vi "Open System Definition.vi"(8 "error in (no error)":errorcluster, 11 "System Definition File":path) -> (0 "error out":errorcluster, 2 "Embedded Data Logger":refnum<k39>, 3 "System Definiton":refnum<k39>)   [LabVIEW 2027, in "Embedded Data Logger Unit Tests.lvclass"]
uses:
  Embedded Data Logger Unit Tests.lvclass
  Embedded Data Logger Unit Tests.lvclass/Embedded Data Logger Unit Tests.ctl
  C:/NetCore/niveristand-embedded-data-logger-custom-device/Source/Tests/Unit/Open System Definition.vi/NationalInstruments.VeriStand.SystemDefinitionAPI
  NationalInstruments.VeriStand.SystemDefinitionAPI
  C:/NetCoreDLL/NationalInstruments.VeriStand.SystemDefinitionAPI.dll
  NetCoreDLL/NationalInstruments.VeriStand.SystemDefinitionAPI.dll
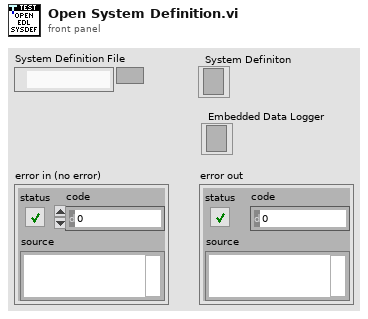
[diagram p1: front panel]
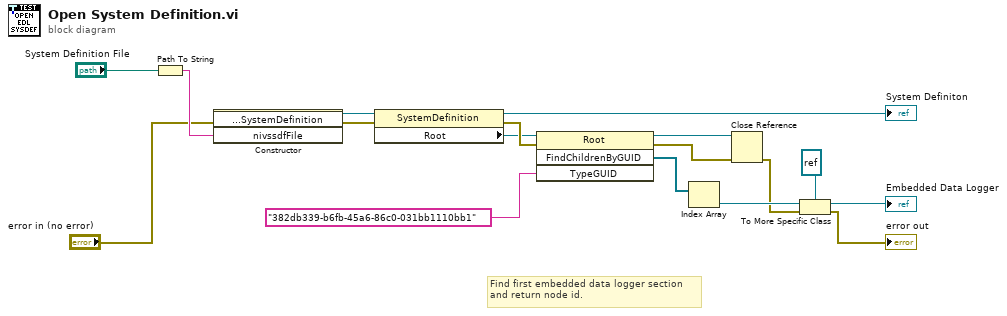
[diagram p0: block diagram]
diagram:
  # "Find first embedded data logger section\nand return node id."
  n1 = Path To String(path="System Definition File") -> (string=w9:string)
  n2 = constructor class="SystemDefinition"(error in="error in (no error)", "nivssdfFile"=w9) -> (reference out=w10:refnum<k39>, error out=w13:errorcluster)  [unwired: 2 in, 2 out]
  n3 = property class="SystemDefinition"(reference=w10, error in=w13) -> (reference out=→"System Definiton":refnum<k39>, error out=w14:errorcluster, "Root"=w11:refnum<k39>)
  n4 = invoke class="Root" method="FindChildrenByGUID"(reference=w11, error in=w14, "TypeGUID"="382db339-b6fb-45a6-86c0-031bb1110bb1") -> (reference out=w15:refnum<k39>, error out=w16:errorcluster, "FindChildrenByGUID"=w12:refnum<k39>[])  [unwired: 1 in, 1 out]
  n5 = Index Array(array=w12) -> (element=w5:refnum<k39>)  [unwired: 1 in]
  n6 = Close Reference(reference=w15, error in (no error)=w16) -> (error out=w4:errorcluster)
  n7 = To More Specific Class(target class=refnum<k39> refnum, reference=w5, error in=w4) -> (specific class reference=→"Embedded Data Logger":refnum<k39>, error out=→"error out":errorcluster)
